vi "TX-SIS-SIM-UDP.vi"() -> ()   [LabVIEW 2018]
uses:
  <vilib>/Platform/TimedLoop/XDataNode/timing_clust.ctl
  <vilib>/Platform/TimedLoop/XDataNode/nitl_modes.ctl
  <vilib>/Platform/TimedLoop/XDataNode/wakeup.ctl
  Global Variables.vi
  <vilib>/Platform/TimedLoop/XDataNode/XDataNode.xnode
  <vilib>/Platform/TimedLoop/XDataNode/XDNodeRunTimeDep.lvlib
panel:
  in  "Stop":bool
  out "BPCS-SIM-TX-ARRAY":dbl[](array[numeric])
  out "length":i32[](array[numeric])
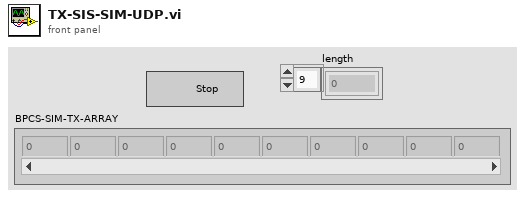
[diagram p1: front panel]
types:
  T1 = typedef "XDNodeRunTimeDep.lvlib/timing_clust.ctl" = cluster{"Expected End [f-1]":u64, "Actual End [f-1]":u64, "Finished Late? [f-1]":bool, "Expected End [i-1]":u64, "Actual End [i-1]":u64, "Finished Late? [i-1]":bool, "Expected Start [i]":u64, "Actual Start [i]":u64, "Expected Start [f]":u64, "Actual Start [f]":u64, "Source Name":string, "Structure Name":string, "Period":i64, "Deadline":i64, "Offset":i64, "Start":i64, "Priority":i32, "Timeout":i32, "Mode":T2, "Wakeup Reason":T3, "Error":errorcluster, "Source Type":string, "Secondary Source Type":string, "Global End Time":u64, "Global Start Time":u64, "Frame Duration":u64, "Iteration Duration":u64, "Assigned CPU":i32, "I/O Scan Engine Mode":u32}
  T2 = typedef "XDNodeRunTimeDep.lvlib/nitl_modes.ctl" = enum32{"No Change", "Process missed periods, maintain original phase", "Discard missed periods, maintain original phase", "Process missed periods, ignore original phase", "Discard missed periods, ignore original phase"}
  T3 = typedef "XDNodeRunTimeDep.lvlib/wakeup.ctl" = enum32{"Normal", "Aborted", "Asynchronous wakeup", "Timing source error", "Timed loop error", "Timeout"}
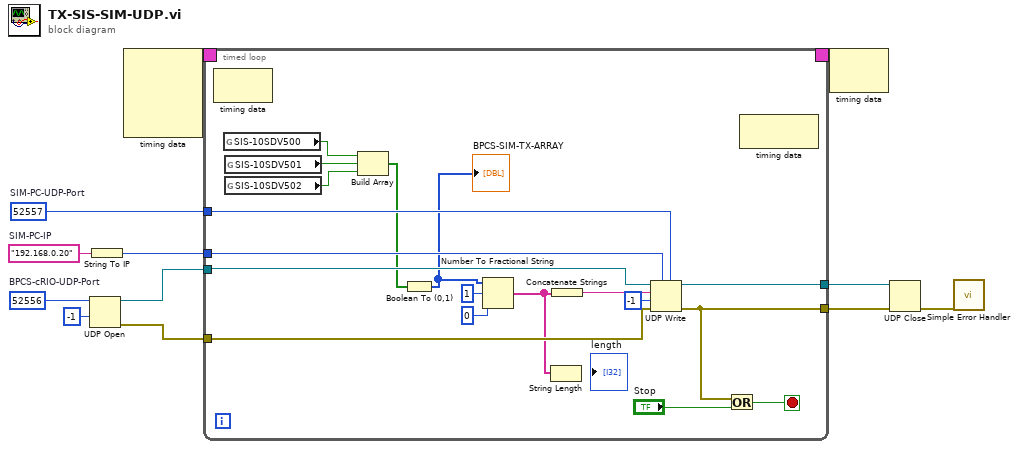
[diagram p0: block diagram]
diagram:
  w7 = u16 52556  # BPCS-cRIO-UDP-Port
  w8 = u16 52557  # SIM-PC-UDP-Port
  w10 = "192.168.0.20"  # SIM-PC-IP
  n1 = UDP Open(9:-1 ("timeout ms (25000)"), 11:w7) -> (port=w6:refnum<k16>, 0:w5:errorcluster)  [unwired: 3 in, 1 out]
  n2 = String To IP(1:w10) -> (0:w9:u32)
  n3 = node-c288() -> (w12:T1)  [unwired: 4 in]
  n4 = timed-loop {
    timing: w12 -> [_]
    timing-out: [_] -> w11
    tunnel: w9 -> [w29]
    tunnel: w8 -> [w28]
    tunnel: w6 -> [w27]
    tunnel: w5 -> [w26]
    tunnel: [w25] -> w4
    tunnel: [w24] -> w3
    stop <- w22 stop-if-true
    n5 = node-c288() -> ()  [unwired: 1 in, 1 out]
    n6 = global read "Global Variables.vi" "SIS-10SDV500"() -> (w16:bool)
    n7 = global read "Global Variables.vi" "SIS-10SDV501"() -> (w14:bool)
    n8 = global read "Global Variables.vi" "SIS-10SDV502"() -> (w15:bool)
    n9 = Build Array(w16, w14, w15) -> (w13:bool[])
    n10 = Boolean To (0,1)(Boolean=w13) -> (0, 1=w18:i16[])
    "BPCS-SIM-TX-ARRAY" <- w18
    n11 = Number To Fractional String(number=w18, width (-)=i16 1, precision (6)=i16 0) -> (F-format string=w21:string[])  [unwired: 1 in]
    n12 = String Length(string=w21) -> ()  [unwired: 1 out]
    n13 = Concatenate Strings(w21) -> (w30:string)
    n14 = UDP Write(address=w29, port or service name=w28, connection ID=w27, data in=w30, 8:w26, 9:-1 ("timeout ms (25000)")) -> (error out=w24:errorcluster, 3:w25:refnum<k16>)
    n15 = Or(x=w24, y="Stop") -> (x .or. y?=w22:bool)
    n16 = node-c288() -> ()  [unwired: 1 in, 1 out]
  }
  n17 = node-c288(w11) -> ()  [unwired: 1 out]
  n18 = UDP Close(connection ID=w4, 8:w3) -> (error out=w2:errorcluster)  [unwired: 1 out]
  n19 = call <vilib>:"Simple Error Handler.vi"("error in (no error)"=w2) -> ()  [unwired: 4 in, 5 out]
